vi "Ramp field.vi"(6 "Error In":errorcluster, 8 "Ramp to set [A/s]":dbl min=0.0 max=0.5, 9 "Field to set [T]":dbl, 10 "PSU Status In":T1 {"Trip Current" format="%.3f"; "Trip Field" format="%.4f"; "Voltage" format="%.2f"; "Field Constant" format="%.6f"; "MID Setpoint (T)" format="%.4f"; "MID Setpoint (A)" format="%.3f"; "MAX Setpoint (T)" format="%.4f"; "MAX Setpoint (A)" format="%.3f"; "Heater Voltage" format="%.2f"; "V Limit (V)" format="%.2f"; "Ramp Rate (A/s)" format="%.3f"; "Output (A)" format="%.3f"; "Output (T)" format="%.4f"; "Persistent Current" format="%.3f"; "Persistent Field" format="%.4f"}, 11 "VISA Refnum in":refnum<visa-resource-name>) -> (0 "error out":errorcluster, 1 "Desired field (T)":dbl, 2 "Ramp Rate (T/s)":dbl, 3 "PSU Status Out":T1 {"Trip Current" format="%.3f"; "Trip Field" format="%.4f"; "Voltage" format="%.2f"; "Field Constant" format="%.6f"; "MID Setpoint (T)" format="%.4f"; "MID Setpoint (A)" format="%.3f"; "MAX Setpoint (T)" format="%.4f"; "MAX Setpoint (A)" format="%.3f"; "Heater Voltage" format="%.2f"; "V Limit (V)" format="%.2f"; "Ramp Rate (A/s)" format="%.3f"; "Output (A)" format="%.3f"; "Output (T)" format="%.4f"; "Persistent Current" format="%.3f"; "Persistent Field" format="%.4f"})   [LabVIEW 2022 SP3, in "Magnet module.lvlib"]
doc: "Set requeiered field and ramp. Then starts ramping.\nReturns status, destination field and ramp rate in T/s."
uses:
  Magnet module.lvlib
  <instrlib>/SMS 120/Public/PSU Status.ctl
  <instrlib>/SMS 120/Cryogenic Ltd SMSXXX.lvlib
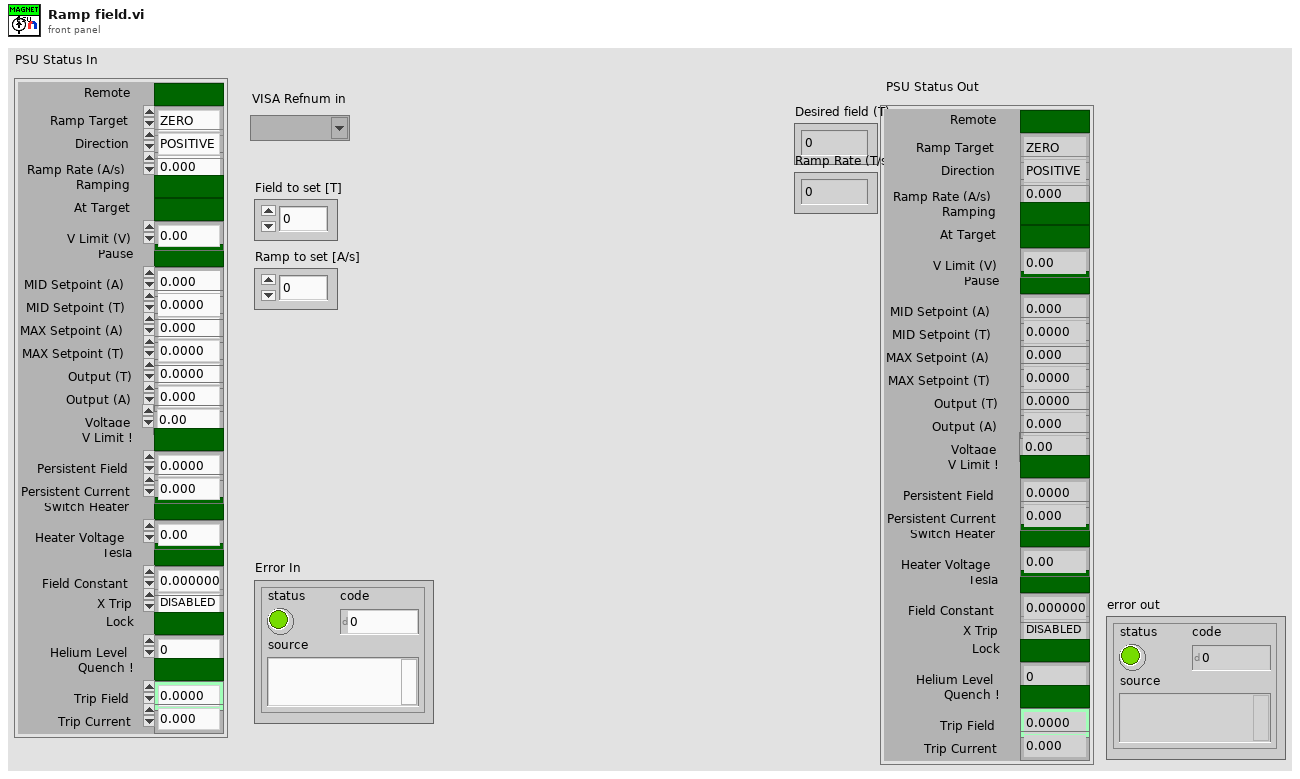
[diagram p1: front panel]
types:
  T1 = typedef "Cryogenic Ltd SMSXXX.lvlib/PSU Status.ctl" = cluster{"Ramp Target":enum16{"ZERO", "MID", "MAX"}, "Pause":bool, "Switch Heater":bool, "Persistent Field":dbl, "Persistent Current":dbl, "Tesla":bool, "Output (T)":dbl, "Output (A)":dbl, "X Trip":enum16{"DISABLED", "ENABLED", "ACTIVE"}, "Ramp Rate (A/s)":dbl, "V Limit (V)":dbl, "Heater Voltage":dbl, "MAX Setpoint (A)":dbl, "MAX Setpoint (T)":dbl, "MID Setpoint (A)":dbl, "MID Setpoint (T)":dbl, "Lock":bool, "Field Constant":dbl, "Remote":bool, "Direction":enum16{"POSITIVE", "NEGATIVE", "OPEN", "UNIPOLAR"}, "Helium Level":u16, "Quench !":bool, "Voltage":dbl, "V Limit !":bool, "Ramping":bool, "At Target":bool, "Trip Field":dbl, "Trip Current":dbl}
  T2 = enum16{"RAMP TO ZERO", "RAMP TO MID", "RAMP TO MAX"}
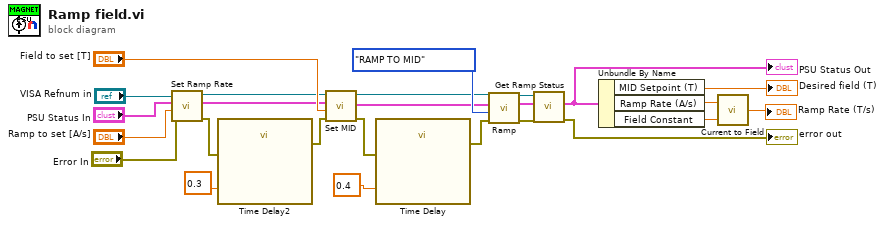
[diagram p0: block diagram]
diagram:
  n1 = call <instrlib>:"Set Ramp Rate.vi"("Error in (no error)"="Error In", "Ramp Rate (A/s)"="Ramp to set [A/s]", "PSU Status In"="PSU Status In", "VISA Resource Name In"="VISA Refnum in") -> ("Error out"=w3:errorcluster, "PSU Status Out"=w13:T1, "VISA Resource Name Out"=w16:refnum<visa-resource-name>)  [unwired: 4 in, 1 out]
  n2 = call "Time Delay2"("error in (no error)"=w3, "Delay Time (s)"=0.3) -> ("error out"=w4:errorcluster)  [unwired: 9 in]
  n3 = call <instrlib>:"Set MID.vi"("Error in (no error)"=w4, "MID (T or A)"="Field to set [T]", "PSU Status In"=w13, "VISA Resource Name In"=w16) -> ("Error out"=w11:errorcluster, "PSU Status Out"=w14:T1, "VISA Resource Name Out"=w15:refnum<visa-resource-name>)  [unwired: 4 in, 1 out]
  n4 = call "Time Delay"("error in (no error)"=w11, "Delay Time (s)"=0.4) -> ("error out"=w10:errorcluster)  [unwired: 9 in]
  n5 = call <instrlib>:"Ramp.vi"("Error in (no error)"=w10, "Ramp Target"=T2."RAMP TO MID", "PSU Status In"=w14, "VISA Resource Name In"=w15) -> ("Error out"=w6:errorcluster, "PSU Status Out"=w8:T1, "VISA Resource Name Out"=w7:refnum<visa-resource-name>)  [unwired: 4 in, 1 out]
  n6 = call <instrlib>:"Get Ramp Status.vi"("Error in (no error)"=w6, "PSU Status In"=w8, "VISA Resource Name In"=w7) -> ("Error out"=→"error out":errorcluster, "PSU Status Out"=w9:T1)  [unwired: 5 in, 2 out]
  "PSU Status Out" <- w9
  n7 = Unbundle By Name(w9) -> ("MID Setpoint (T)"=→"Desired field (T)":dbl, "Ramp Rate (A/s)"=w22:dbl, "Field Constant"=w21:dbl)
  n8 = call "Current to Field.vi"("Field constant [T/A]"=w21, "Current in [A]"=w22) -> ("Field out [T]"=→"Ramp Rate (T/s)":dbl)
